vi "RS-485 Transceiver Control.vi"() -> ()   [LabVIEW 2023]
doc: "This example sets the RS-485 transceiver control modes for the specified port and performs a serial port read, a serial port write, or a combination of these actions. If all are selected, the VI will write the data first, read data and then close the VISA session that is opened to the port. This VI will wait until the specified number of bytes is received at the port or until a termination character is received. This example will work only with National Instruments RS-485 interfaces.\n\nThis example demonstrates the transceiver control modes available when using a National Instruments RS-485 product. When connecting one or several devices via RS-485, a user may want to cut down on the amount of wiring. Alternatively, some devices offer a certain wiring configuration that you may need to match. Determine the wiring needs of the connected serial device to determine which NI RS-485 transceiver control mode to choose.\n\nWhen you are communicating with a two-wire device, National Instruments recommends that you use the two-wire Auto Control mode. This mode handles the transmitter/receiver enabling for a two-wire connection in your hardware, so it reduces the software overhead required to perform this operation in your application program."
uses:
  support/Serial - Settings.ctl
  <vilib>/Instr/_visa.llb/VISA Configure Serial Port (Instr).vi
panel:
  in  "Termination Character":u8=10 format="%.0x"
  in  "End Write on Termination Character?":bool=TRUE
  in  "End Read on Termination Character?":bool=TRUE
  in  "RS-485 Transceiver Mode":u16(ring) items=["Wire4", "Wire2-EchoDTR", "Wire2-CtrlDTR", "Wire2-Auto"]
  in  "Write String":string="*IDN?"
  in  "Serial Settings":T1={"baud rate"=9600, "data bits"=8, "parity"=enum."None", "stop bits"=10, "flow control"=0} {"flow control" items=["None"=0, "XON/XOFF"=1, "RTS/CTS"=2, "DTR/DSR"=4]; "stop bits" items=["1.0"=10, "1.5"=15, "2.0"=20]; "data bits" min=5 max=8 step=1; "baud rate" items=["75"=75, "110"=110, "134"=134, "150"=150, "300"=300, "600"=600, "1200"=1200, "1800"=1800, "2400"=2400, "4800"=4800, "7200"=7200, "9600"=9600, "14400"=14400, "19200"=19200, "28800"=28800, "38400"=38400, "56000"=56000, "57600"=57600, "115200"=115200, "128000"=128000, "230400"=230400]}
  in  "Assert DTR?":bool
  out "Response":string
  in  "VISA RS 485 Resource":refnum<visa-resource-name>="COM1"
  # "Overview: Demonstrates the use of the VISA functions to configure NI RS-485 hardware.\nRequirements: NI-Serial and NI-VISA Drivers, NI RS-485 hardware\nInstructions:\n1. Ensure the resource specified in the VISA RS 485 Resource control is a valid NI RS-485 device, and that the Assert DTR? value is correct for your device.\n2. Specify the proper RS-485 Transceiver Mode value for your device.\n3. Run the VI.\n4. View the Response returned by the device."
  # "0xA is equivalent to a '\\n' character, which is a line feed."
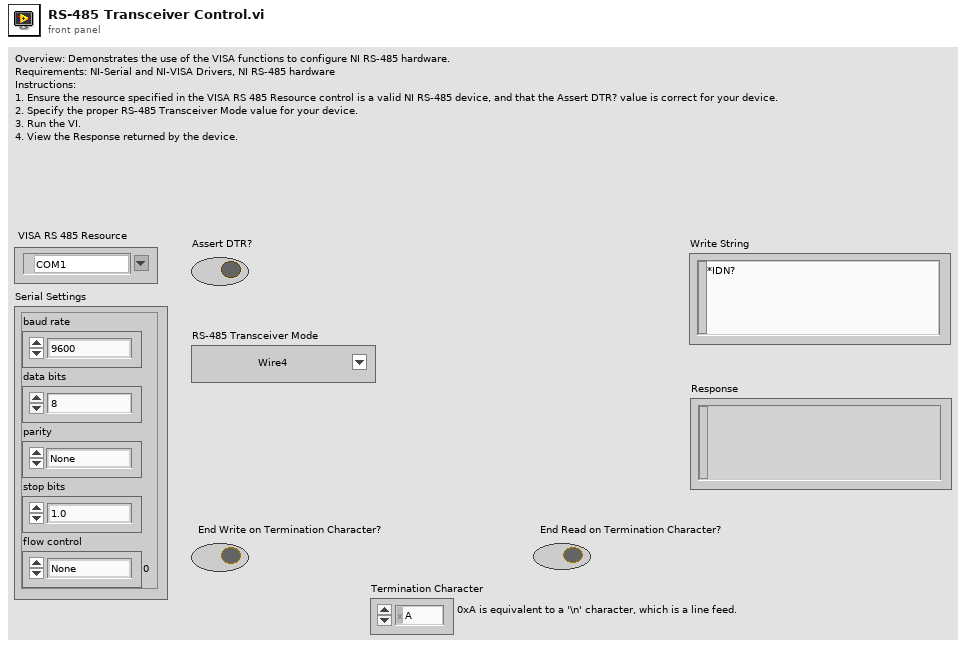
[diagram p1: front panel]
types:
  T1 = typedef "Serial - Settings.ctl" = cluster{"baud rate":u32, "data bits":u16, "parity":enum16{"None", "Odd", "Even", "Mark", "Space"}, "stop bits":u16, "flow control":u16}
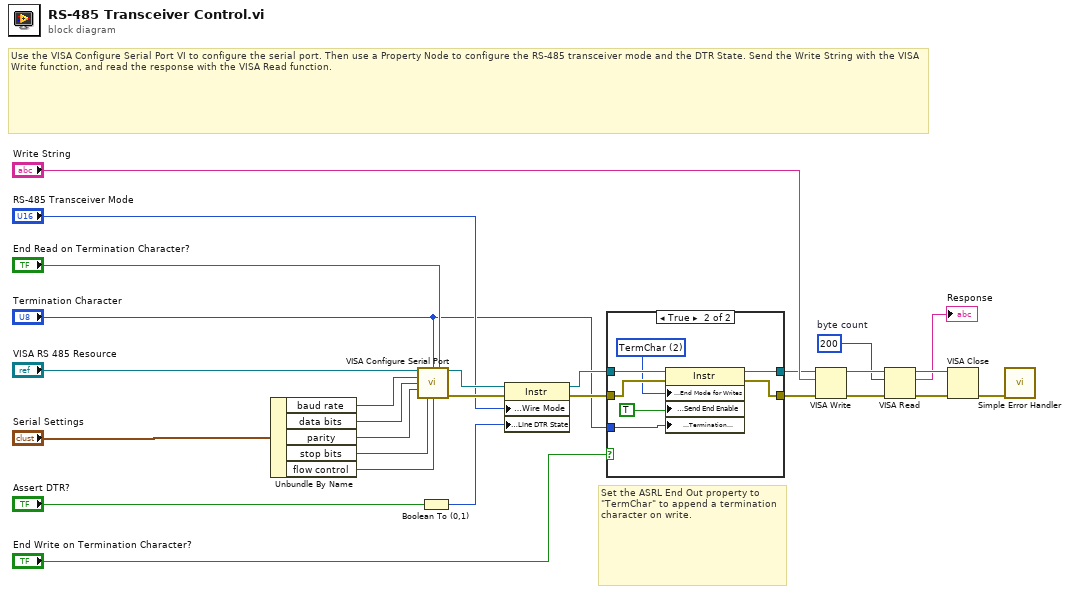
[diagram p0: block diagram]
diagram:
  w17 = u32 200  # byte count
  # "Set the ASRL End Out property to \"TermChar\" to append a termination character on write."
  # "Use the VISA Configure Serial Port VI to configure the serial port. Then use a Property Node to configure the RS-485 transceiver mode and the DTR State. Send the Write String with the VISA Write function, and read the response with the VISA Read function."
  n1 = Unbundle By Name("Serial Settings") -> ("baud rate"=w14:u32, "data bits"=w13:u16, "parity"=w12:enum16{"None", "Odd", "Even", "Mark", "Space"}, "stop bits"=w11:u16, "flow control"=w10:u16)
  n2 = call-poly "VISA Configure Serial Port"("VISA resource name"="VISA RS 485 Resource", "termination char\n(0xA = '\\n' = LF)"="Termination Character", "Enable Termination\nChar (T)"="End Read on Termination Character?", "baud rate (9600)"=w14, "data bits (8)"=w13, "parity (0:none)"=w12, "stop bits (10: 1 bit)"=w11, "flow control (0:none)"=w10) -> ("VISA resource name out"=w23:refnum<visa-resource-name>, "error out"=w22:errorcluster)  [unwired: 2 in, 4 out]
  n3 = Boolean To (0,1)(Boolean="Assert DTR?") -> (0, 1=w20:i16)
  n4 = property class="Instr"(reference=w23, error in=w22, "Serial Settings:Wire Mode"="RS-485 Transceiver Mode", "Serial Settings:Modem Line Settings:Line DTR State"=w20) -> (reference out=w4:refnum<visa-resource-name>, error out=w5:errorcluster)
  n5 = case shown="True" "End Write on Termination Character?" {
    tunnel: w4 -> [w28 w36]
    tunnel: w5 -> [w29 w35]
    tunnel: [w28 w34] -> w3
    tunnel: [w29 w33] -> w6
    tunnel: "Termination Character" -> [_ w31]
    frame False {
    }
    frame True {
      w32 = u16 2 items=["None", "LastBit", "TermChar", "Break"] ("Serial Settings:Serial End Mode for Writes")
      n6 = property class="Instr"(reference=w36, error in=w35, "Serial Settings:End Mode for Writes"=w32, "Message Based Settings:Send End Enable"=TRUE, "Message Based Settings:Termination Character"=w31) -> (reference out=w34:refnum<visa-resource-name>, error out=w33:errorcluster)
    }
  }
  n7 = VISA Write(VISA resource name=w3, write buffer="Write String", error in (no error)=w6) -> (VISA resource name out=w26:refnum<visa-resource-name>, error out=w19:errorcluster)  [unwired: 1 out]
  n8 = VISA Read(VISA resource name=w26, byte count=w17, error in (no error)=w19) -> (VISA resource name out=w24:refnum<visa-resource-name>, read buffer=→"Response":string, error out=w25:errorcluster)  [unwired: 1 out]
  n9 = VISA Close(VISA resource name=w24, error in (no error)=w25) -> (error out=w18:errorcluster)
  n10 = call <vilib>:"Simple Error Handler.vi"("error in (no error)"=w18) -> ()  [unwired: 1 in, 8 out]
